vi "MS-2000 Read Positions.vi"(7 "WHERE Reply":string=" ", 11 "Error In":errorcluster) -> (4 "Positions um":dbl[](array[numeric]), 8 "Success":bool, 15 "Error Out":errorcluster)   [LabVIEW 2020]
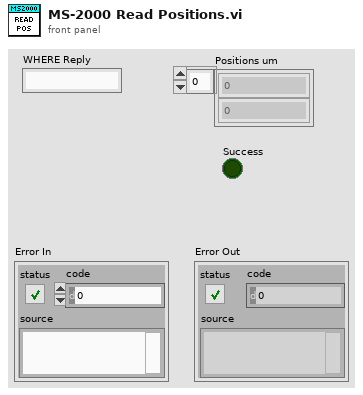
[diagram p1: front panel]
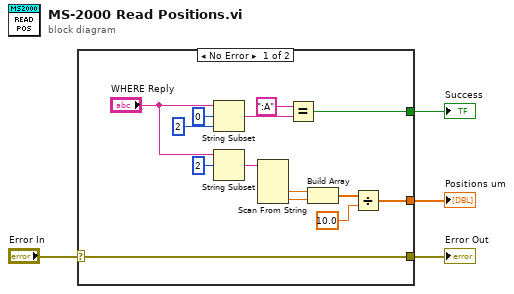
[diagram p0: block diagram]
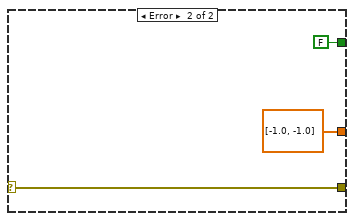
[diagram p2: hidden frame]
diagram:
  n1 = case shown="No Error" "Error In" {
    selector: "Error In" -> [w5 w19]
    tunnel: [w12 FALSE] -> w4
    tunnel: [w7 dbl[] [-1.0, -1.0]] -> w3
    tunnel: [w5 w19] -> w1
    frame No Error {
      n2 = String Subset(string="WHERE Reply", offset (0)=0, length (rest)=2 ("length (rest)")) -> (substring=w14:string)
      n3 = String Subset(string="WHERE Reply", offset (0)=2) -> (substring=w15:string)  [unwired: 1 in]
      n4 = Scan From String(input string=w15) -> (output 1=w11:dbl, output 2=w10:dbl)  [unwired: 5 in, 3 out]
      n5 = Equal?(x=":A", y=w14) -> (x = y?=w12:bool)
      n6 = Build Array(w11, w10) -> (w9:dbl[])
      n7 = Divide(x=w9, y=10.0) -> (x/y=w7:dbl[])
    }
    frame Error {
    }
  }
  "Success" <- w4
  "Positions um" <- w3
  "Error Out" <- w1
